vi "Start Test Explorer.vi"(6 "Variant in":variant, 7 "Shift Pressed?":bool, 8 "error in (no error)":errorcluster, 10 "QD Combo Box Ref":refnum<vi>, 11 "QD Launch VI Ref":refnum<vi>) -> (0 "error out":errorcluster, 4 "Variant out":variant)   [LabVIEW 2017]
doc: "Launches Test Explorer.\n\nDefault Shortcut - [E]"
uses:
  Test Explorer/Test Explorer.vi
  Test Explorer/Test Explorer.lvlib
panel:
  in  "Undo Name":string="Start Test Explorer (LVUnit)"
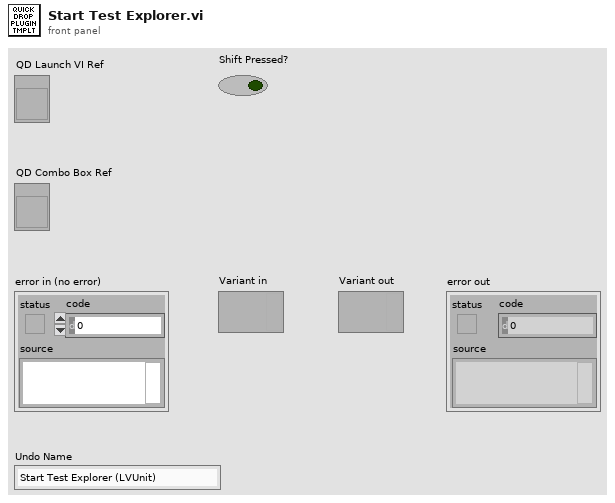
[diagram p1: front panel]
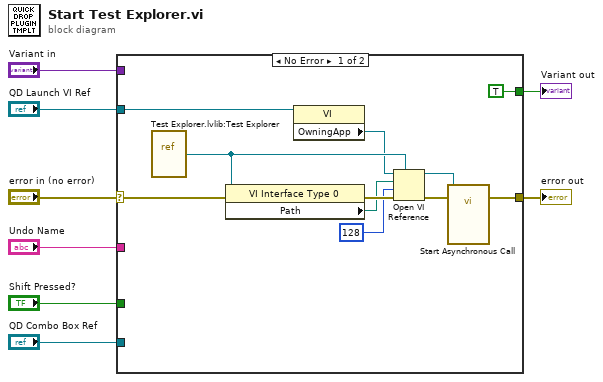
[diagram p0: block diagram]
diagram:
  n1 = case shown="No Error" "error in (no error)" {
    selector: "error in (no error)" -> [w14 w20]
    tunnel: [w12 w20] -> w7
    tunnel: "QD Launch VI Ref" -> [w10 _]
    tunnel: "Shift Pressed?" -> [_ _]
    tunnel: "QD Combo Box Ref" -> [_ _]
    tunnel: "Variant in" -> [_ _]
    tunnel: "Undo Name" -> [_ _]
    tunnel: [TRUE _] -> w1
    frame No Error {
      n2 = vi-ref "Test Explorer.lvlib:Test Explorer.vi"() -> (w16:refnum<vi>)
      n3 = property class="VI Interface Type 0"(reference=w16, error in=w14) -> (error out=w17:errorcluster, "Path"=w15:path)  [unwired: 1 out]
      n4 = property class="VI"(reference=w10) -> ("OwningApp"=w9:refnum<vi>)  [unwired: 1 in, 2 out]
      n5 = Open VI Reference(type specifier VI Refnum (for type only)=w16, application reference (local)=w9, vi path=w15, options=128, error in (no error)=w17) -> (vi reference=w11:refnum<vi>, error out=w18:errorcluster)  [unwired: 1 in]
      n6 = call-by-ref "Start Asynchronous Call"(reference=w11, error in=w18) -> (error out=w12:errorcluster)  [unwired: 12 in, 1 out]
    }
    frame Error {
    }
  }
  "error out" <- w7
  "Variant out" <- w1
